vi "get_value.vi"(8 "error in (no error)":errorcluster, 11 "OpResult in":refnum<class "OpResult.lvclass">) -> (0 "error out":errorcluster, 2 "mlir.lvlib:SsaId.lvclass":refnum<class "SsaId.lvclass">, 3 "OpResult out":refnum<class "OpResult.lvclass">)   [LabVIEW 2020, in "mlir.lvlib" / "OpResult.lvclass"]
uses:
  OpResult.lvclass
  OpResult.lvclass/OpResult.ctl
  SsaId/SsaId.lvclass
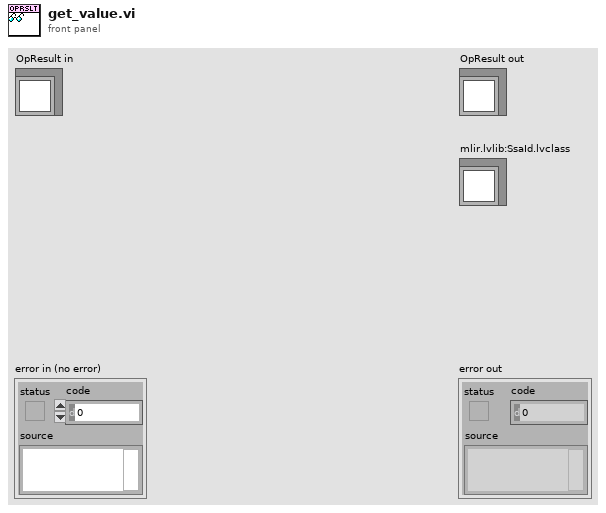
[diagram p1: front panel]
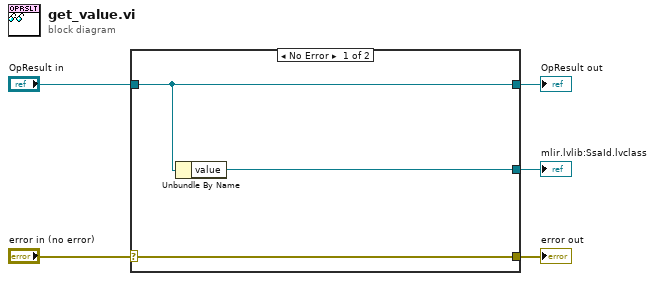
[diagram p0: block diagram]
diagram:
  n1 = case shown="No Error" "error in (no error)" {
    selector: "error in (no error)" -> [w8 w9]
    tunnel: [w8 w9] -> w4
    tunnel: [w7 w10] -> w2
    tunnel: "OpResult in" -> [w7 w10]
    tunnel: [w6 _] -> w1
    frame No Error {
      n2 = Unbundle By Name(w7) -> ("value"=w6:refnum<class "SsaId.lvclass">)
    }
    frame Error {
    }
  }
  "error out" <- w4
  "OpResult out" <- w2
  "mlir.lvlib:SsaId.lvclass" <- w1
